vi "Generate Firmware Interface Config Message.vi"(8 "Error In":errorcluster, 9 "Device Type":u16(ring) items=["chipKIT Uno32", "chipKIT uC32", "chipKIT Max32", "chipKIT DP32"], 10 "Device Family":u16(ring) items=["National Instruments", "Digilent", "Arduino"], 11 "Firmware Program Interface":u16(ring) items=["Serial / USB"]) -> (0 "Error Out":errorcluster, 3 "Config Message":string)   [LabVIEW 2013, in "LVH-LINX.lvlib"]
uses:
  <vilib>/LabVIEW Hacker/LINX/LVH-LINX.lvlib
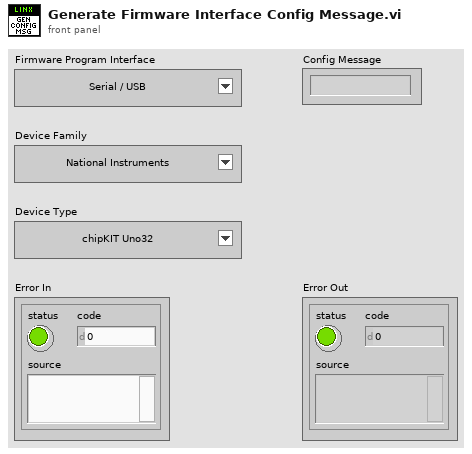
[diagram p1: front panel]
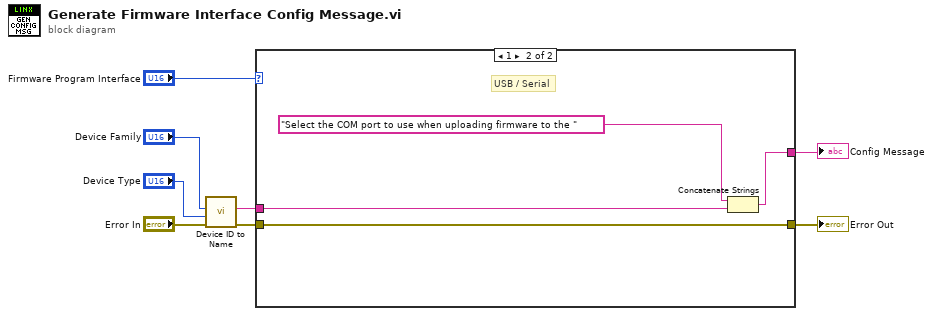
[diagram p0: block diagram]
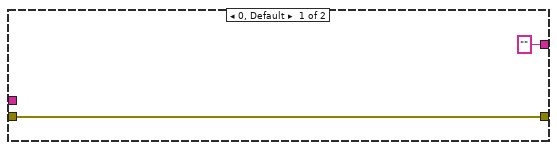
[diagram p2: hidden frame]
diagram:
  n1 = call <vilib>:"Device ID to Name.vi"("Error In"="Error In", "Device ID"="Device Type", "Device Family"="Device Family") -> ("Error Out"=w2:errorcluster, "Device Name"=w1:string)  [unwired: 6 in, 1 out]
  n2 = case shown="1" "Firmware Program Interface" {
    tunnel: w2 -> [w10 w12]
    tunnel: [w10 w12] -> w7
    tunnel: ["" w13] -> w6
    tunnel: w1 -> [_ w11]
    frame 0, Default {
    }
    frame 1 {
      # "USB / Serial"
      n3 = Concatenate Strings("Select the COM port to use when uploading firmware to the ", w11) -> (w13:string)
    }
  }
  "Error Out" <- w7
  "Config Message" <- w6
